vi "SCD - wavelenght.vi"(11 "SCD Emission Line Filter":T1) -> (3 "Numeric":dbl)   [LabVIEW 2014]
uses:
  Controls/SCD - EDT - Emission Line Filter Wheel.ctl
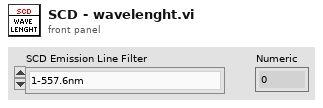
[diagram p1: front panel]
types:
  T1 = typedef "SCD - EDT - Emission Line Filter Wheel.ctl" = enum16{"1-557.6nm", "2-587.6nm", "3-589.6nm", "4-630.2nm", "5-656.4nm", "6-849.8nm", "7-854.2nm", "8-866.2nm", "9-1083.0nm"}
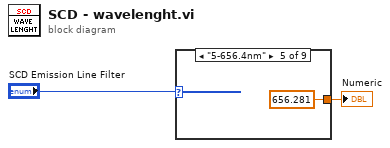
[diagram p0: block diagram]
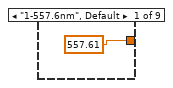
[diagram p2: hidden frame]
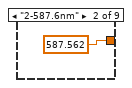
[diagram p3: hidden frame]
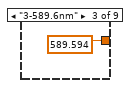
[diagram p4: hidden frame]
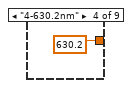
[diagram p5: hidden frame]
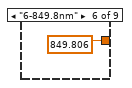
[diagram p6: hidden frame]
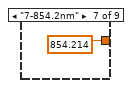
[diagram p7: hidden frame]
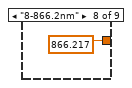
[diagram p8: hidden frame]
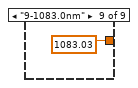
[diagram p9: hidden frame]
diagram:
  n1 = case shown="\"5-656.4nm\"" "SCD Emission Line Filter" {
    tunnel: [557.61 587.562 589.594 630.2 656.281 849.806 854.214 866.217 1083.03] -> w2
    frame "1-557.6nm", Default {
    }
    frame "2-587.6nm" {
    }
    frame "3-589.6nm" {
    }
    frame "4-630.2nm" {
    }
    frame "5-656.4nm" {
    }
    frame "6-849.8nm" {
    }
    frame "7-854.2nm" {
    }
    frame "8-866.2nm" {
    }
    frame "9-1083.0nm" {
    }
  }
  "Numeric" <- w2
